vi "NIIE_Const Temp Coordinate 4 points.vi"() -> (3 "Const Temp Coordinate":T1={"Horizontal"=-10000, "Vertical"=-10000, "Vertical 2"=-10000, "Vertical 3"=-10000})   [LabVIEW 2021]
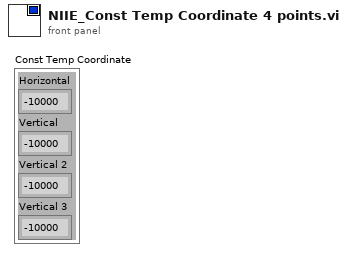
[diagram p1: front panel]
types:
  T1 = cluster{"Horizontal":i32, "Vertical":i32, "Vertical 2":i32, "Vertical 3":i32}
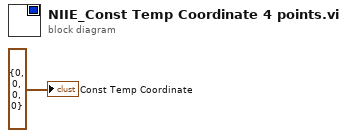
[diagram p0: block diagram]
diagram:
  "Const Temp Coordinate" <- T1 {"Horizontal"=0, "Vertical"=0, "Vertical 2"=0, "Vertical 3"=0} ("Temp Coord")
